vi "Sample_01.vi"() -> ()   [LabVIEW 2018]
uses:
  <vilib>/Instr/_visa.llb/VISA Configure Serial Port (Instr).vi
panel:
  in  "VISA resource name 2":refnum<visa-resource-name>="COM5"
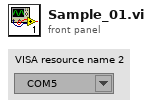
[diagram p1: front panel]
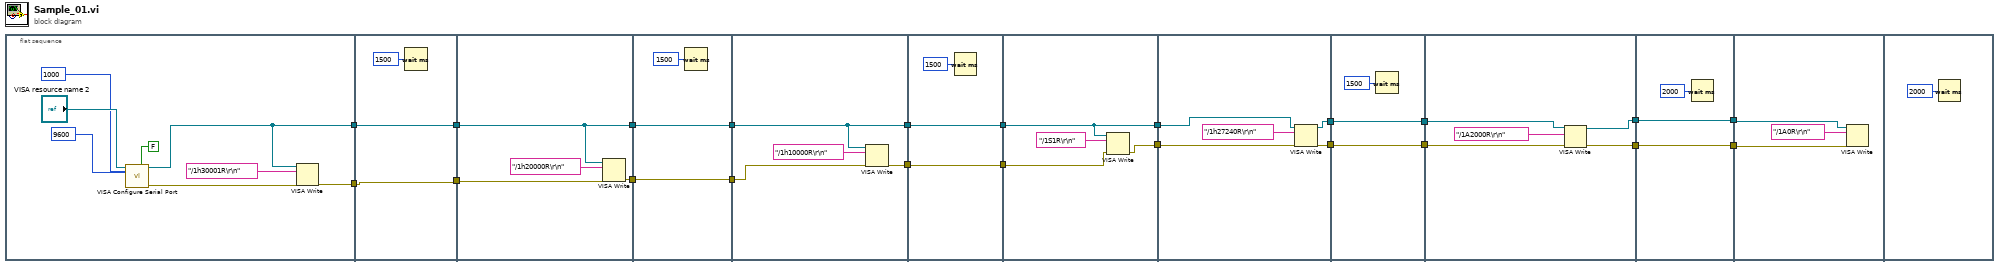
[diagram p0: block diagram]
diagram:
  n1 = flat-sequence {
    tunnel: [w25] -> w22
    tunnel: [w24] -> w21
    tunnel: w22 -> [w32]
    tunnel: w21 -> [w31]
    tunnel: [w32] -> w20
    tunnel: [w31] -> w19
    tunnel: w20 -> [w35]
    tunnel: w19 -> [w36]
    tunnel: [w35] -> w17
    tunnel: [w34] -> w15
    tunnel: [w39] -> w18
    tunnel: w17 -> [w39]
    tunnel: [w38] -> w16
    tunnel: w15 -> [w38]
    tunnel: w18 -> [w41]
    tunnel: w16 -> [w43]
    tunnel: [w42] -> w13
    tunnel: [w41] -> w11
    tunnel: [w46] -> w14
    tunnel: w13 -> [w46]
    tunnel: w11 -> [w45]
    tunnel: [w45] -> w10
    tunnel: w14 -> [w50]
    tunnel: [w49] -> w12
    tunnel: w10 -> [w48]
    tunnel: [w48] -> w9
    tunnel: w12 -> [w55]
    tunnel: w9 -> [w54]
    tunnel: [w53] -> w7
    tunnel: [w52] -> w5
    tunnel: [w58] -> w8
    tunnel: w7 -> [w58]
    tunnel: [w57] -> w6
    tunnel: w5 -> [w57]
    tunnel: w8 -> [w63]
    tunnel: w6 -> [w62]
    tunnel: [w61] -> w3
    tunnel: [w60] -> w1
    tunnel: [w66] -> w4
    tunnel: w3 -> [w66]
    tunnel: [w65] -> w2
    tunnel: w1 -> [w65]
    tunnel: w4 -> [w69]
    tunnel: w2 -> [w68]
    frame #0 {
      n2 = call-poly "VISA Configure Serial Port"("VISA resource name"="VISA resource name 2", "timeout (10sec)"=u32 1000, "Enable Termination\nChar (T)"=FALSE ("Enable Termination\nChar (T)"), "baud rate (9600)"=u32 9600) -> ("VISA resource name out"=w25:refnum<visa-resource-name>, "error out"=w26:errorcluster)  [unwired: 10 in]
      n3 = VISA Write(VISA resource name=w25, write buffer="/1h30001R\r\n" ("string"), error in (no error)=w26) -> (error out=w24:errorcluster)  [unwired: 2 out]
    }
    frame #1 {
      n4 = Wait (ms)(milliseconds to wait=u32 1500) -> ()  [unwired: 1 out]
    }
    frame #2 {
      n5 = VISA Write(VISA resource name=w35, write buffer="/1h20000R\r\n" ("string"), error in (no error)=w36) -> (error out=w34:errorcluster)  [unwired: 2 out]
    }
    frame #3 {
      n6 = Wait (ms)(milliseconds to wait=u32 1500) -> ()  [unwired: 1 out]
    }
    frame #4 {
      n7 = VISA Write(VISA resource name=w41, write buffer="/1h10000R\r\n" ("string"), error in (no error)=w43) -> (error out=w42:errorcluster)  [unwired: 2 out]
    }
    frame #5 {
      n8 = Wait (ms)(milliseconds to wait=u32 1500) -> ()  [unwired: 1 out]
    }
    frame #6 {
      n9 = VISA Write(VISA resource name=w48, write buffer="/1S1R\r\n" ("string"), error in (no error)=w50) -> (error out=w49:errorcluster)  [unwired: 2 out]
    }
    frame #7 {
      n10 = VISA Write(VISA resource name=w54, write buffer="/1h27240R\r\n" ("string"), error in (no error)=w55) -> (VISA resource name out=w52:refnum<visa-resource-name>, error out=w53:errorcluster)  [unwired: 1 out]
    }
    frame #8 {
      n11 = Wait (ms)(milliseconds to wait=u32 1500) -> ()  [unwired: 1 out]
    }
    frame #9 {
      n12 = VISA Write(VISA resource name=w62, write buffer="/1A2000R\r\n" ("string"), error in (no error)=w63) -> (VISA resource name out=w60:refnum<visa-resource-name>, error out=w61:errorcluster)  [unwired: 1 out]
    }
    frame #10 {
      n13 = Wait (ms)(milliseconds to wait=u32 2000) -> ()  [unwired: 1 out]
    }
    frame #11 {
      n14 = VISA Write(VISA resource name=w68, write buffer="/1A0R\r\n" ("string"), error in (no error)=w69) -> ()  [unwired: 3 out]
    }
    frame #12 {
      n15 = Wait (ms)(milliseconds to wait=u32 2000) -> ()  [unwired: 1 out]
    }
  }
